vi "ADVM_IntermodulationDistortion_POC.vi"() -> ()   [LabVIEW 2021]
uses:
  <vilib>/PDM Acquisition Toolkit/host/Classes/Tasks/PDM Tasks/Controls/Acquisition Mode.ctl
  <vilib>/addons/_NISVFA/_Generation/Signal Generation/SV Signal/sv_System Timing Model.ctl
  <vilib>/PDM Acquisition Toolkit/shared/controls/PCM Data Format Configuration.ctl
  <vilib>/PDM Acquisition Toolkit/shared/controls/Digital Edge.ctl
  <vilib>/PDM Acquisition Toolkit/shared/controls/PCM Bit Endianness.ctl
  <vilib>/PDM Acquisition Toolkit/shared/controls/PCM Data Justification.ctl
  <vilib>/PDM Acquisition Toolkit/shared/controls/PCM Frame Sync Control.ctl
  <vilib>/PDM Acquisition Toolkit/host/Classes/Session/Controls/Logic Levels.ctl
  <vilib>/PDM Acquisition Toolkit/host/Classes/Tasks/PDM Tasks/PDM Task.lvclass
  <vilib>/PDM Acquisition Toolkit/host/Classes/Tasks/PCM Input/Controls/DVR PCM Input Task.ctl
  <vilib>/PDM Acquisition Toolkit/host/Classes/Tasks/PCM Input/PCM Input Task.lvclass
  <vilib>/DAQmx/write.llb/DAQmx Write (Analog 1D Wfm NChan NSamp).vi
  <vilib>/addons/_NISVFA/_Shared subVIs/Common/SVL Set dB Reference (1 Ch).vi
  <vilib>/addons/_NISVFA/_Shared subVIs/Common/SVL Set dB Reference (variant).vi
  <vilib>/addons/_NISVFA/_Generation/Signal Generation/SV Multitone/SV Multitone.lvclass
  C:/Program Files/National Instruments/LabVIEW 2021/vi.lib/addons/_NISVFA/_Generation/Signal Generation/SV Signal/SV Signal.lvclass
  <vilib>/DAQmx/create/channels.llb/DAQmx Create Channel (AO-Voltage-Basic).vi
  <vilib>/DAQmx/configure/timing.llb/DAQmx Timing (Sample Clock).vi
  <vilib>/addons/_NISVFA/_Generation/Signal Generation/SV Multitone/Configure Multitone (Custom).vi
  <vilib>/addons/_NISVFA/_Generation/Signal Generation/SV Signal/Write Sample Rate.vi
  <vilib>/addons/_NISVFA/_Generation/Signal Generation/SV Signal/Write System Timing Model.vi
  <vilib>/addons/_NISVFA/_Generation/Signal Generation/SV Signal/Write Ramp Parameters.vi
  <vilib>/DAQmx/miscellaneous.llb/DAQmx Fill In Error Info.vi
  <vilib>/PDM Acquisition Toolkit/host/API/Public/Create Tasks/Create PCM Input Task.vi
  <vilib>/PDM Acquisition Toolkit/host/API/Public/Configure/Timing/Configure Timing - PCM Input Slave.vi
  <vilib>/PDM Acquisition Toolkit/host/API/Public/Configure/PDM Channel/Configure Microphone Sensitivity FSPA - PCM Input Task.vi
  <vilib>/PDM Acquisition Toolkit/host/API/Public/Utility/Configure Simulation Mode.vi
  <vilib>/PDM Acquisition Toolkit/host/API/Public/Start/Start PDM Task.vi
  <vilib>/PDM Acquisition Toolkit/host/API/Public/Read/Read PCM Input Waveform.vi
  <vilib>/addons/_NISVFA/_Shared subVIs/Common/svc_Caller VI Returned in Error Source.vi
  <vilib>/addons/Sound and Vibration/svt_Distortion/SVT Intermodulation Distortion (1 Ch).vi
  <vilib>/PDM Acquisition Toolkit/host/API/Public/Clear/Clear PCM Input Task.vi
  <vilib>/PDM Acquisition Toolkit/host/API/PDM Acquisition Toolkit.lvlib
  <vilib>/addons/Sound and Vibration/svt_Distortion/SoundVib_Distortion.lvlib
  <vilib>/addons/_NISVFA/_Generation/Signal Generation/SV Signal/SV Signal.lvclass
  <resource>/objmgr/daqmx.rc
  <vilib>/PDM Acquisition Toolkit/shared/PDM Shared.lvlib
  <vilib>/PDM Acquisition Toolkit/host/Classes/Session/DecoderSession.lvclass
panel:
  out "error out":errorcluster
  in  "Tab Control 3":enum32{"Analog Source", "Protocol Settings"}(tab)
  in  "DAQmx Physical Channel":tag="PXI1Slot3/ao0"
  in  "Amplitude":dbl=-1.0 format="%#_g dB"
  in  "IMD standard":T1(ring)=enum."CCIF (11 kHz, 12 kHz, 1:1)"
  in  "Custom IMD Signal":T2={"low-frequency tone"=14000.0, "high-frequency tone"=15000.0, "amplitude ratio"=1.0} {"amplitude ratio" format="%.1f"; "high-frequency tone" format="%.2f"; "low-frequency tone" format="%.2f"}
  in  "Resource Name":string="7821\\PCMi 0"
  in  "Number of words":i32=19200
  in  "Data latch at SCK cycle":u8=50 min=50 max=140 format="%.0f%"
  in  "Bit Clock rate (Hz)":u32=2822400 format="%.4p"
  out "IMD (dB)":dbl format="%.2f"
  in  "Tab Control 2":enum32{"Frequency Domain", "Time Domain"}(tab)
  out "Spectrum":cluster{"x0":dbl, "dx":dbl, "magnitude":dbl[]}(graph)={"x0"=0.0, "dx"=1.0, "magnitude"=[]}
  out "Time Domain":waveform(dbl)[](graph)
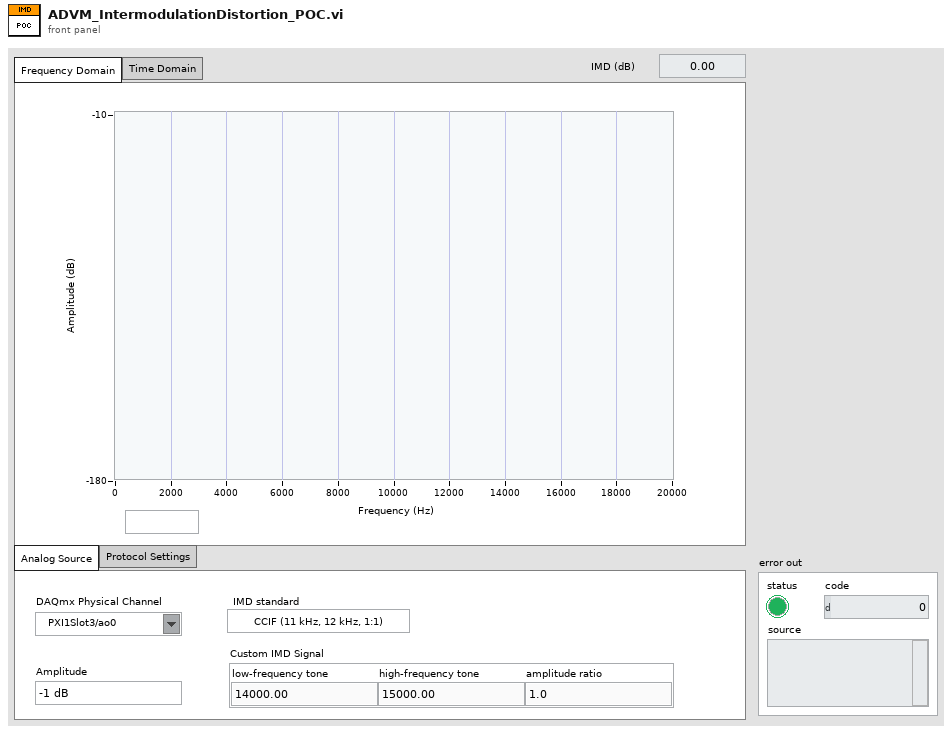
[diagram p1: front panel]
types:
  T1 = enum16{"SMPTE (60 Hz, 7000 Hz, 4:1)", "DIN (250 Hz, 8000 Hz, 4:1)", "CCIF (11 kHz, 12 kHz, 1:1)", "CCIF (19 kHz, 20 kHz, 1:1)", "Custom"}
  T2 = cluster{"low-frequency tone":dbl, "high-frequency tone":dbl, "amplitude ratio":dbl}
  T3 = typedef "PDM Acquisition Class Library.lvlib/PCM Input Task.lvclass/DVR PCM Input Task.ctl" = refnum<data-value>
  T4 = typedef "PDM Acquisition Class Library.lvlib/DecoderSession.lvclass/Logic Levels.ctl" = enum16{"3.3 V", "1.8 V", "1.2 V"}
  T5 = typedef "PDM Shared.lvlib/PCM Frame Sync Control.ctl" = cluster{"Frame Length":u16, "Frame Sync Pulse Width":u16, "Bit Clock Edge  Sync":T6}
  T6 = typedef "PDM Shared.lvlib/Digital Edge.ctl" = enum8{"Rising", "Falling"}
  T7 = typedef "PDM Shared.lvlib/PCM Data Format Configuration.ctl" = cluster{"Frame Sync Edge for Channel 0":T6, "Channel Count Per Frame":u8, "Channel Length":u16, "Bit Depth":u8, "Channel 0 Offset":u16, "Endianness":T8, "Data Justification":T9}
  T8 = typedef "PDM Shared.lvlib/PCM Bit Endianness.ctl" = enum16{"MSB First", "LSB First"}
  T9 = typedef "PDM Shared.lvlib/PCM Data Justification.ctl" = enum16{"Left Justified", "Right Justified"}
  T10 = cluster{"IMD type":enum16{"SMPTE/DIN", "CCIF/Twin-Tone"}, "low-frequency tone":dbl, "high-frequency tone":dbl, "amplitude ratio":dbl, "maximum order":i32}
  T11 = cluster{"profile":enum16{"Linear", "Half cosine"}, "durations [s]":cluster{"ramp-up":dbl, "transition":dbl, "ramp-down":dbl}}
  T12 = typedef "SV Signal.lvclass/sv_System Timing Model.ctl" = i64
  T13 = cluster{"IMD units":enum16{"dB", "linear ratio", "%"}, "intermodulation component amplitude units":enum16{"EU rms", "EU peak", "EU peak-peak"}, "detected fundamental amplitude units":enum16{"EU rms", "EU peak", "EU peak-peak"}, "magnitude spectrum units":enum16{"dB", "linear"}}
  T14 = typedef "PDM Acquisition Class Library.lvlib/PDM Task.lvclass/Acquisition Mode.ctl" = enum16{"Finite", "Continuous"}
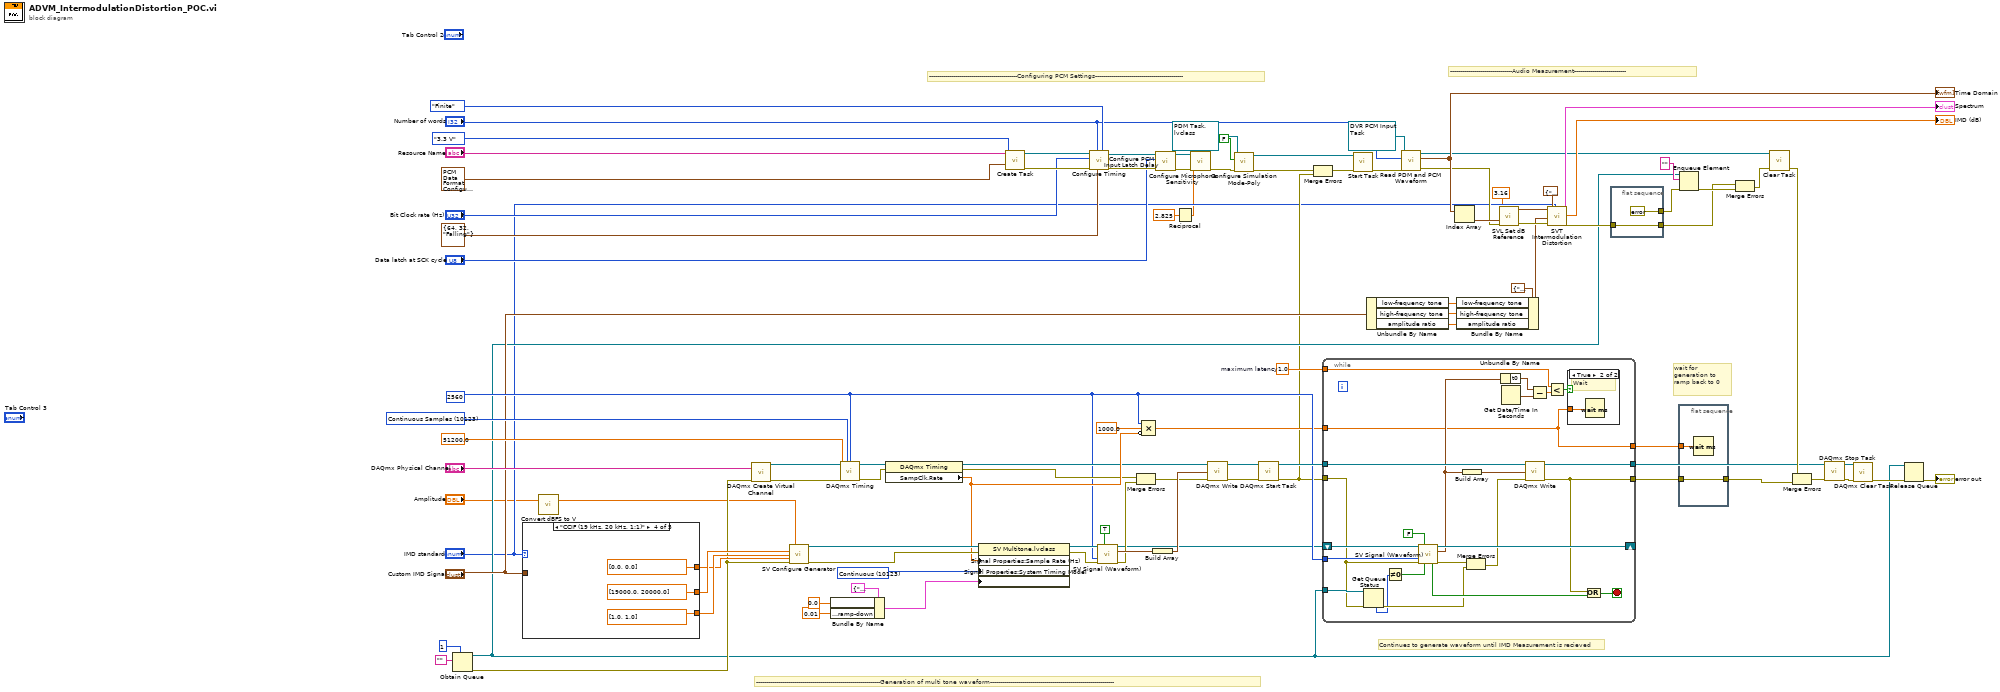
[diagram p0: block diagram]
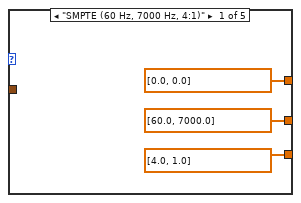
[diagram p2: hidden frame]
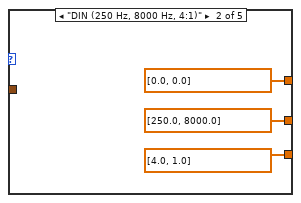
[diagram p3: hidden frame]
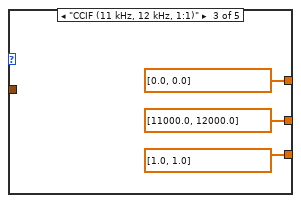
[diagram p4: hidden frame]
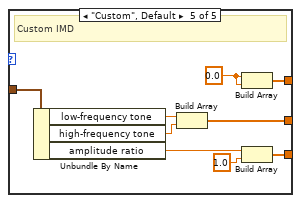
[diagram p5: hidden frame]
diagram:
  w41 = 1.0  # maximum latency
  w58 = T12 10123 items=["Finite"=10178, "-"=-1, "Continuous"=10123, "-"=-2, "Settled"=110123, "Averaged"=210123, "Discrete Sweep"=310123, "Continuous Sweep"=410123] ("System Timing Model")
  w37 = 2560 ("samples per channel")
  w63 = 10123 items=["Finite Samples"=10178, "Continuous Samples"=10123, "Hardware Timed Single Point"=12522] ("sample mode")
  # "Continues to generate waveform until IMD Measurement is recieved"
  # "-------------------------------Audio Measurement--------------------------"
  # "--------------------------------------------------------------Generation of multi tone waveform--------------------------------------------------------------"
  # "--------------------------------------------Configuring PCM Settings--------------------------------------------"
  # "wait for generation to ramp back to 0"
  n1 = Obtain Queue(max queue size (-1, unlimited)=1, element data type="") -> (queue out=w27:refnum<queue>, error out=w67:errorcluster)  [unwired: 3 in, 1 out]
  n2 = case shown="\"CCIF (19 kHz, 20 kHz, 1:1)\"" "IMD standard" {
    tunnel: "Custom IMD Signal" -> [_ _ _ _ w120]
    tunnel: [dbl[] [60.0, 7000.0] ("source settings.frequencies") dbl[] [250.0, 8000.0] ("source settings.frequencies") dbl[] [11000.0, 12000.0] ("source settings.frequencies") dbl[] [19000.0, 20000.0] ("source settings.frequencies") w114] -> w71
    tunnel: [dbl[] [4.0, 1.0] ("source settings.frequencies") dbl[] [4.0, 1.0] ("source settings.frequencies") dbl[] [1.0, 1.0] ("source settings.frequencies") dbl[] [1.0, 1.0] ("source settings.frequencies") w113] -> w70
    tunnel: [dbl[] [0.0, 0.0] ("source settings.frequencies") dbl[] [0.0, 0.0] ("source settings.frequencies") dbl[] [0.0, 0.0] ("source settings.frequencies") dbl[] [0.0, 0.0] ("source settings.frequencies") w112] -> w69
    frame "SMPTE (60 Hz, 7000 Hz, 4:1)" {
    }
    frame "DIN (250 Hz, 8000 Hz, 4:1)" {
    }
    frame "CCIF (11 kHz, 12 kHz, 1:1)" {
    }
    frame "CCIF (19 kHz, 20 kHz, 1:1)" {
    }
    frame "Custom", Default {
      w115 = 0.0 ("element")
      # "Custom IMD"
      n3 = Unbundle By Name(w120) -> ("low-frequency tone"=w119:dbl, "high-frequency tone"=w118:dbl, "amplitude ratio"=w117:dbl)
      n4 = Build Array(w119, w118) -> (w114:dbl[])
      n5 = Build Array(w115, w115) -> (w112:dbl[])
      n6 = Build Array(w117, 1.0 ("element")) -> (w113:dbl[])
    }
  }
  n7 = call "Convert dBFS to V.vi"("Amplitude dBFS"="Amplitude") -> ("Amplitude V"=w9:dbl)  [unwired: 2 in]
  n8 = call-poly <vilib>:"DAQmx Create Virtual Channel.vi"("physical channels"="DAQmx Physical Channel", "error in"=w67) -> ("task out"=w65:refnum<k21>, "error out"=w66:errorcluster)  [unwired: 12 in]
  n9 = call-poly <vilib>:"SV Configure Generator.vi"("overall amplitude"=w9, "frequencies [Hz]"=w71, "amplitudes"=w70, "phases [deg]"=w69, "error in (no error)"=w67) -> ("signal configuration"=w60:refnum<class "SV Multitone.lvclass">, "error out"=w59:errorcluster)  [unwired: 8 in, 1 out]
  n10 = Bundle By Name(cluster=T11 {"profile"=enum."Linear", "durations [s]"={"ramp-up"=0.0, "transition"=0.0, "ramp-down"=0.0}} ("Ramp Parameters:All Elements"), "durations [s].ramp-up"=0.0, "durations [s].ramp-down"=0.01) -> (w54:T11)
  n11 = call-poly <vilib>:"DAQmx Timing.vi"("task/channels in"=w65, "sample mode"=w63, "samples per channel"=w37, "rate"=51200.0, "error in"=w66) -> ("task out"=w61:refnum<k21>, "error out"=w62:errorcluster)  [unwired: 9 in]
  n12 = property class="DAQmx Timing"(reference=w61, error in=w62) -> (reference out=w43:refnum<k21>, error out=w46:errorcluster, "SampClk.Rate"=w50:dbl)
  n13 = property class="SV Multitone.lvclass"(reference=w60, error in=w59, "Signal Properties:Sample Rate (Hz)"=w50, "Signal Properties:System Timing Model"=w58, "Signal Properties:Ramps:Ramp Parameters"=w54) -> (reference out=w53:refnum<class "SV Multitone.lvclass">, error out=w52:errorcluster)
  n14 = call-poly <vilib>:"Create Task.vi"("PCM data configuration"=T7 {"Frame Sync Edge for Channel 0"=enum."Falling", "Channel Count Per Frame"=2, "Channel Length"=32, "Bit Depth"=24, "Channel 0 Offset"=1, "Endianness"=enum."MSB First", "Data Justification"=enum."Left Justified"}, "logic level"=Logic_Levels."3.3 V", "channel list"="Resource Name") -> ("error out"=w98:errorcluster, "PCM input task out"=w96:T3)  [unwired: 7 in]
  n15 = call-poly <vilib>:"Configure Timing.vi"("acquisition mode"=Acquisition_Mode."Finite", "Frame Sync Clock Control"=T5 {"Frame Length"=64, "Frame Sync Pulse Width"=32, "Bit Clock Edge  Sync"=enum."Falling"}, "number of words per channel"="Number of words", "error in"=w98, "Bit Clock rate"="Bit Clock rate (Hz)", "PCM input task in"=w96) -> ("error out"=w22:errorcluster, "PCM input task out"=w21:T3)  [unwired: 4 in]
  n16 = call-dynamic "SV Signal (Waveform).vi"("signal configuration"=w53, "reset"=TRUE, "samples"=w37, "error in (no error)"=w52) -> ("signal configuration"=w25:refnum<class "SV Multitone.lvclass">, "output waveform"=w48:waveform(dbl), "error out"=w47:errorcluster)  [unwired: 6 in, 3 out]
  n17 = Merge Errors(w46, w47) -> (w6:errorcluster)
  n18 = Compound Arithmetic op=MULTIPLY(w37, 1000.0 ("value"), invert w50) -> (w36:dbl)
  n19 = Build Array(w48) -> (w45:waveform(dbl)[])
  n20 = call <vilib>:"Configure PCM Input Latch Delay.vi"("error in"=w22, "Latch Delay(ns)"="Data latch at SCK cycle", "PCM input task in"=w21) -> ("error out"=w18:errorcluster, "PCM input task out"=w19:T3)  [unwired: 6 in, 1 out]
  n21 = Reciprocal(x=2.825 ("microphone sensitivity (FS/Pa)")) -> (1/x=w3:dbl)
  n22 = call-poly <vilib>:"Configure Microphone Sensitivity.vi"("error in"=w18, "microphone sensitivity (FS/Pa)"=w3, "PCM input task in"=w19) -> ("error out"=w16:errorcluster)  [unwired: 7 in, 1 out]
  n23 = call-poly <vilib>:"DAQmx Write.vi"("task/channels in"=w43, "data"=w45, "error in"=w6) -> ("task out"=w44:refnum<k21>, "error out"=w42:errorcluster)  [unwired: 10 in, 1 out]
  n24 = call-poly <vilib>:"Configure Simulation Mode-Poly.vi"("error in"=w16, "simulation mode"=FALSE, "PDM input task in"=refnum<data-value> refnum) -> ("error out"=w15:errorcluster, "PDM input task out"=w17:refnum<data-value>)  [unwired: 7 in]
  n25 = call <vilib>:"DAQmx Start Task.vi"("task/channels in"=w44, "error in"=w42) -> ("task out"=w38:refnum<k21>, "error out"=w26:errorcluster)  [unwired: 12 in]
  n26 = Merge Errors(w15, w26) -> (w95:errorcluster)
  n27 = while {
    tunnel: w26 -> [w125]
    shift-right: [w143] -> _
    shift-left: w25 -> [w144]
    tunnel: w37 -> [w132]
    tunnel: w38 -> [w140]
    tunnel: [w139] -> w34
    tunnel: [w138] -> w39
    tunnel: w41 -> [w134]
    tunnel: w36 -> [w122]
    tunnel: w27 -> [w127]
    tunnel: [w122] -> w40
    stop <- w142 stop-if-true
    n28 = Get Queue Status(queue=w127, error in (no error)=w125) -> (error out=w124:errorcluster, # elements in queue=w123:i32)  [unwired: 1 in, 6 out]
    n29 = Not Equal To 0?(x=w123) -> (x != 0?=w126:bool)
    n30 = call-dynamic "SV Signal (Waveform).vi"("signal configuration"=w144, "reset"=FALSE, "samples"=w132, "error in (no error)"=w125, "stop"=w126) -> ("signal configuration"=w143:refnum<class "SV Multitone.lvclass">, "output waveform"=w131:waveform(dbl), "done"=w141:bool, "error out"=w129:errorcluster)  [unwired: 5 in, 2 out]
    n31 = Build Array(w131) -> (w130:waveform(dbl)[])
    n32 = Merge Errors(w129, w124) -> (w128:errorcluster)
    n33 = Unbundle By Name(w131) -> ("t0"=w137:timestamp)
    n34 = Get Date/Time In Seconds() -> (seconds since 1Jan1904=w136:timestamp)
    n35 = call-poly <vilib>:"DAQmx Write.vi"("task/channels in"=w140, "data"=w130, "error in"=w128) -> ("task out"=w139:refnum<k21>, "error out"=w138:errorcluster)  [unwired: 10 in, 1 out]
    n36 = Subtract(x=w137, y=w136) -> (x-y=w135:dbl)
    n37 = Less?(x=w134, y=w135) -> (x < y?=w133:bool)
    n38 = case shown="True" w133 {
      tunnel: w122 -> [_ w145]
      frame False {
      }
      frame True {
        # "Wait"
        n39 = Wait (ms)(milliseconds to wait=w145) -> ()  [unwired: 1 out]
      }
    }
    n40 = Or(x=w138, y=w141) -> (x .or. y?=w142:bool)
  }
  n41 = call-poly <vilib>:"Start Task.vi"("error in"=w95, "PDM input task in"=w17) -> ("error out"=w97:errorcluster)  [unwired: 8 in, 1 out]
  n42 = Unbundle By Name("Custom IMD Signal") -> ("low-frequency tone"=w33:dbl, "high-frequency tone"=w32:dbl, "amplitude ratio"=w31:dbl)
  n43 = call-poly <vilib>:"Read PDM and PCM Waveform.vi"("error in"=w97, "words per channel"="Number of words", "PCM input task In"=T3 refnum) -> ("error out"=w91:errorcluster, "PCM waveforms"=w94:waveform(dbl)[], "PCM input task out"=w79:T3)  [unwired: 3 in, 3 out]
  "Time Domain" <- w94
  n44 = Index Array(array=w94) -> (element=w92:waveform(dbl))  [unwired: 1 in]
  n45 = Bundle By Name(cluster=T10 {"IMD type"=enum."CCIF/Twin-Tone", "low-frequency tone"=14000.0, "high-frequency tone"=15000.0, "amplitude ratio"=1.0, "maximum order"=5} ("custom IMD signal"), "low-frequency tone"=w33, "high-frequency tone"=w32, "amplitude ratio"=w31) -> (w29:T10)
  n46 = call-poly <vilib>:"SVL Set dB Reference.vi"("error in (no error)"=w91, "dB reference [EU]"=3.16, "scaled signal in [EU]"=w92) -> ("error out"=w89:errorcluster, "scaled signal out [EU]"=w90:waveform(dbl))  [unwired: 7 in]
  n47 = call-poly <vilib>:"SVT Intermodulation Distortion.vi"("scaled signal [EU]"=w90, "custom IMD signal"=w29, "error in"=w89, "desired units"=T13 {"IMD units"=enum."dB", "intermodulation component amplitude units"=enum."EU rms", "detected fundamental amplitude units"=enum."EU rms", "magnitude spectrum units"=enum."dB"}, "IMD standard"="IMD standard") -> ("magnitude spectrum"=→"Spectrum":cluster{"f0":dbl, "df":dbl, "magnitude":dbl[]}, "IMD"=→"IMD (dB)":dbl, "error out"=w80:errorcluster)  [unwired: 7 in, 5 out]
  n48 = flat-sequence {
    tunnel: w80 -> [w146]
    tunnel: [errorcluster {"status"=FALSE, "code"=0, "source"=""} ("error in (no error)")] -> w83
    tunnel: [w146] -> w81
    frame #0 {
    }
  }
  n49 = flat-sequence {
    tunnel: w40 -> [w149]
    tunnel: w39 -> [w148]
    tunnel: [w148] -> w35
    frame #0 {
      n50 = Wait (ms)(milliseconds to wait=w149) -> ()  [unwired: 1 out]
    }
  }
  n51 = Enqueue Element(queue=w27, element="", error in (no error)=w83) -> (error out=w82:errorcluster)  [unwired: 1 in, 2 out]
  n52 = Merge Errors(w81, w82) -> (w78:errorcluster)
  n53 = call-poly <vilib>:"Clear Task.vi"("error in"=w78, "PCM input task in"=w79) -> ("error out"=w72:errorcluster)  [unwired: 9 in]
  n54 = Merge Errors(w72, w35) -> (w74:errorcluster)
  n55 = call <vilib>:"DAQmx Stop Task.vi"("task/channels in"=w34, "error in"=w74) -> ("task out"=w76:refnum<k21>, "error out"=w75:errorcluster)  [unwired: 12 in]
  n56 = call <vilib>:"DAQmx Clear Task.vi"("task in"=w76, "error in"=w75) -> ("error out"=w73:errorcluster)  [unwired: 13 in]
  n57 = Release Queue(queue=w27, error in (no error)=w73) -> (error out=→"error out":errorcluster)  [unwired: 1 in, 2 out]
